vi "ElevatorSim_UpdateX.vi"(8 "dT_Seconds":dbl=1.0, 9 "U":T4, 10 "current_xHat":T4, 11 "ELEVATOR_SIM":T1 {"GearBox"."Kt_NMPerAmp" format="%13.5p"; "GearBox"."Kv_RadPerSecPerVolt" format="%13.5p"; "GearBox"."R_Ohms" format="%13.5p"; "GearBox"."FreeSpeed_RadPerSec" format="%13.5p"; "GearBox"."FreeCurrent_Amps" format="%13.5p"; "GearBox"."StallCurrent_Amps" format="%13.5p"; "GearBox"."StallTorque_NM" format="%13.5p"; "GearBox"."nominalVoltage_Volts" format="%13.5p"}) -> (3 "updated_xHat":T4)   [LabVIEW 2019, in "Trajectory_Library.lvlib"]
doc: "Creates a new LINEAR SYSTEM data cluster with the specified values. \n\n\nInputs: \n - XXX -- XXX.\n\nOutputs:\n - XXX -- XXX."
uses:
  Trajectory_Library.lvlib
  <vilib>/Analysis/Matrix/Datatypes/RealMatrix.ctl
  ELEVATOR_SIM.ctl
  LINEAR_SYSTEM_SIM.ctl
  LINEAR_SYSTEM.ctl
  DCMOTOR.CTL
  MatBuilder_Create.vi
  ElevatorSim_Rkf45_Func.vi
  <vilib>/Analysis/Matrix/NI_Matrix.lvlib
panel:
  # "<States, 1>"
  # "<Outputs, 1>"
  # "<Inputs, 1>"
  # "<Outputs, 1>"
  # "<States,States>"
  # "<States,Inputs>"
  # "<Outputs,States>"
  # "<Outputs,Inputs>"
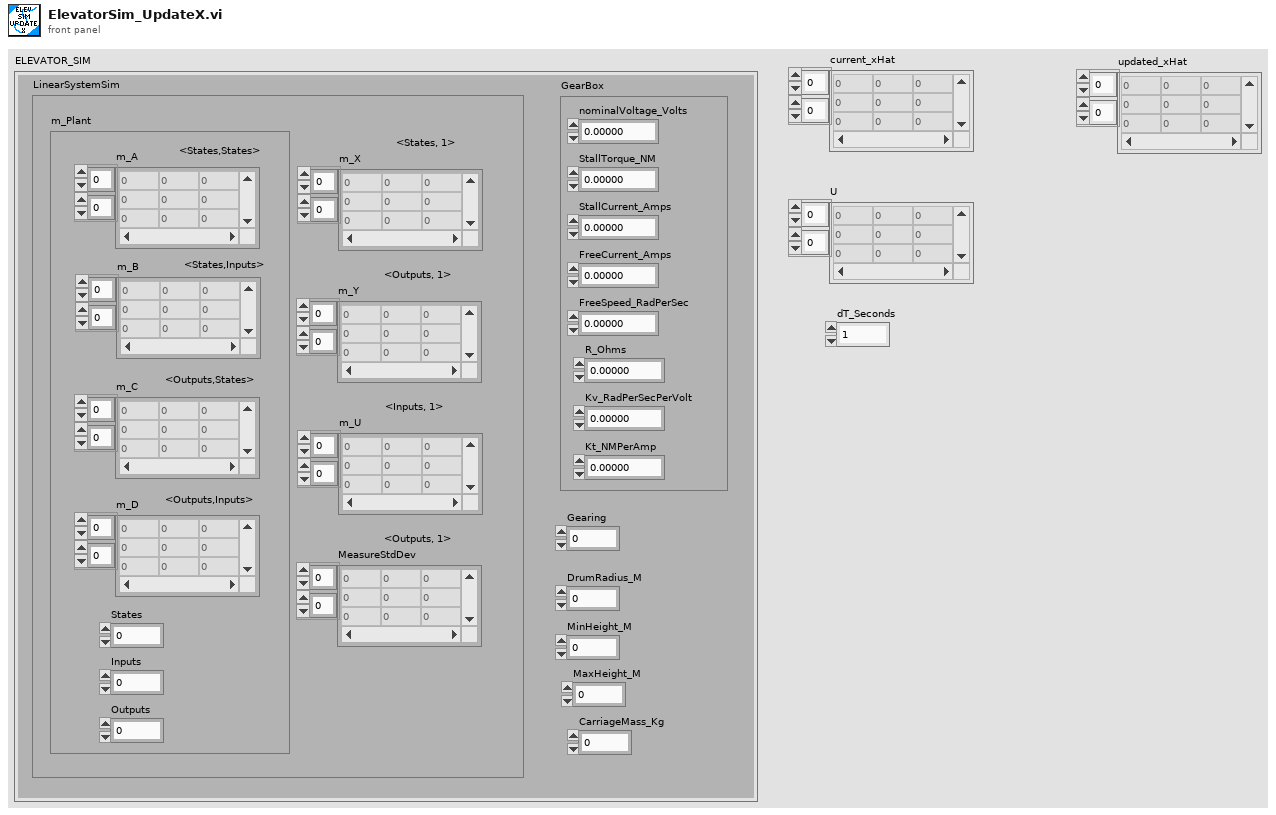
[diagram p1: front panel]
types:
  T1 = typedef "Trajectory_Library.lvlib/ELEVATOR_SIM.ctl" = cluster{"LinearSystemSim":T2, "GearBox":T5, "Gearing":dbl, "DrumRadius_M":dbl, "MinHeight_M":dbl, "MaxHeight_M":dbl, "CarriageMass_Kg":dbl}
  T2 = typedef "Trajectory_Library.lvlib/LINEAR_SYSTEM_SIM.ctl" = cluster{"m_Plant":T3, "m_X":T4, "m_Y":T4, "m_U":T4, "MeasureStdDev":T4}
  T3 = typedef "Trajectory_Library.lvlib/LINEAR_SYSTEM.ctl" = cluster{"m_A":T4, "m_B":T4, "m_C":T4, "m_D":T4, "States":i32, "Inputs":i32, "Outputs":i32}
  T4 = typedef "NI_Matrix.lvlib/RealMatrix.ctl" = dbl[][]
  T5 = typedef "Trajectory_Library.lvlib/DCMOTOR.CTL" = cluster{"nominalVoltage_Volts":dbl, "StallTorque_NM":dbl, "StallCurrent_Amps":dbl, "FreeCurrent_Amps":dbl, "FreeSpeed_RadPerSec":dbl, "R_Ohms":dbl, "Kv_RadPerSecPerVolt":dbl, "Kt_NMPerAmp":dbl}
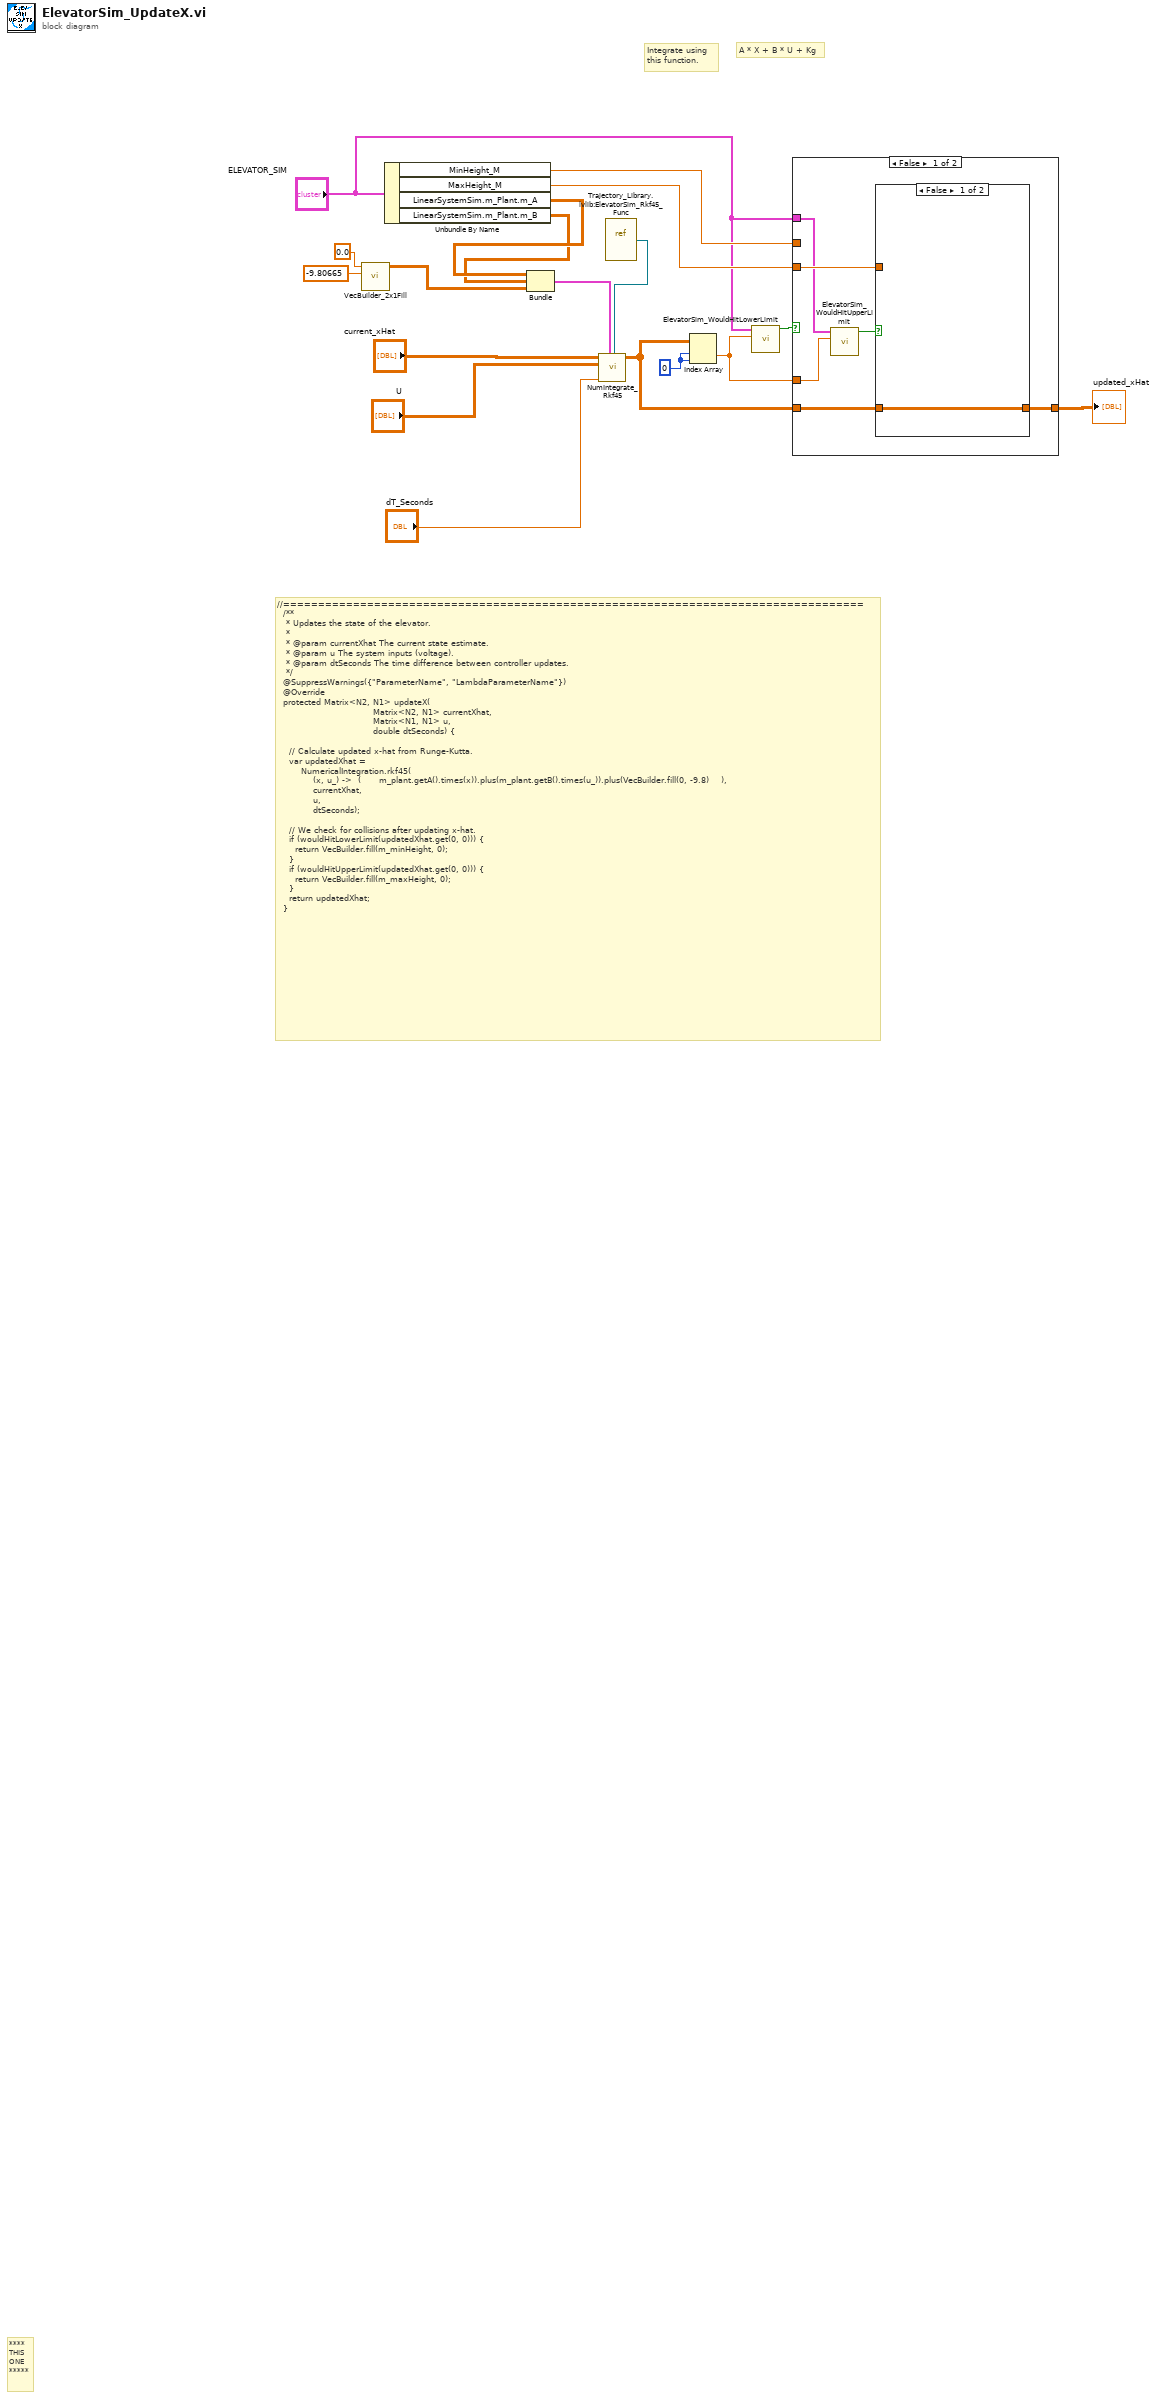
[diagram p0: block diagram]
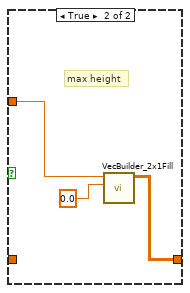
[diagram p2: hidden frame]
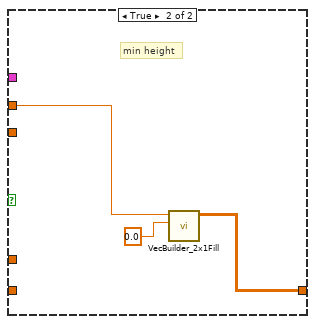
[diagram p3: hidden frame]
diagram:
  w13 = 0 ("index (row)")
  # "Integrate using\nthis function."
  # "A * X + B * U + Kg"
  # "//===================================================================================\n  /**\n   * Updates the state of the elevator.\n   *\n   * @param currentXhat The current state estimate.\n   * @param u The system inputs (voltage).\n   * @param dtSeconds The time difference between controller updates.\n   */\n  @SuppressWarnings({\"ParameterName\", \"LambdaParameterName\"})\n  @Override\n  protected Matrix<N2, N1> updateX(\n                                Matrix<N2, N1> currentXhat, \n                                Matrix<N1, N1> u, \n                                double dtSeconds) {\n\n    // Calculate updated x-hat from Runge-Kutta.\n    var updatedXhat =\n        NumericalIntegration.rkf45(\n            (x, u_) ->  (      m_plant.getA().times(x)).plus(m_plant.getB().times(u_)).plus(VecBuilder.fill(0, -9.8)    ),\n            currentXhat,\n            u,\n            dtSeconds);\n\n    // We check for collisions after updating x-hat.\n    if (wouldHitLowerLimit(updatedXhat.get(0, 0))) {\n      return VecBuilder.fill(m_minHeight, 0);\n    }\n    if (wouldHitUpperLimit(updatedXhat.get(0, 0))) {\n      return VecBuilder.fill(m_maxHeight, 0);\n    }\n    return updatedXhat;\n  }"
  # "****\nTHIS\nONE\n*****"
  n1 = call "VecBuilder_2x1Fill.vi"("R1"=-9.80665, "R0"=0.0) -> ("output matrix"=w3:T4)  [unwired: 9 in]
  n2 = Unbundle By Name("ELEVATOR_SIM") -> ("MinHeight_M"=w7:dbl, "MaxHeight_M"=w12:dbl, "LinearSystemSim.m_Plant.m_A"=w5:T4, "LinearSystemSim.m_Plant.m_B"=w4:T4)
  n3 = Bundle("m_A"=w5, "m_B"=w4, "output matrix"=w3) -> (w2:cluster{"m_A":T4, "m_B":T4, "output matrix":T4})  [unwired: 1 in]
  n4 = vi-ref "Trajectory_Library.lvlib:ElevatorSim_Rkf45_Func.vi"() -> (w1:refnum<vi>)
  n5 = call "NumIntegrate_Rkf45.vi"("NumInt_RKF45_Func_Type"=w1, "PassedData"=w2, "dT_Seconds"="dT_Seconds", "U"="U", "X"="current_xHat") -> ("Return X"=w11:T4)  [unwired: 5 in, 1 out]
  n6 = Index Array(array=w11, index (row)=w13, index (col)=w13) -> (element=w8:dbl)
  n7 = call "ElevatorSim_WouldHitLowerLimit.vi"("ElevHeight_Meters"=w8, "ElevatorSim"="ELEVATOR_SIM") -> ("AtLowLimit"=w9:bool)  [unwired: 9 in]
  n8 = case shown="False" w9 {
    tunnel: w12 -> [w20 _]
    tunnel: w11 -> [w24 _]
    tunnel: [w23 w29] -> w10
    tunnel: w8 -> [w21 _]
    tunnel: w7 -> [_ w30]
    tunnel: "ELEVATOR_SIM" -> [w19 _]
    frame False {
      n9 = call "ElevatorSim_WouldHitUpperLimit.vi"("Height_Meters"=w21, "ElevatorSim"=w19) -> ("At HIgh LImit"=w22:bool)  [unwired: 9 in]
      n10 = case shown="False" w22 {
        tunnel: w24 -> [w25 _]
        tunnel: [w25 w26] -> w23
        tunnel: w20 -> [_ w27]
        frame False {
        }
        frame True {
          # "max height"
          n11 = call "VecBuilder_2x1Fill.vi"("R1"=0.0, "R0"=w27) -> ("output matrix"=w26:T4)  [unwired: 9 in]
        }
      }
    }
    frame True {
      # "min height"
      n12 = call "VecBuilder_2x1Fill.vi"("R1"=0.0, "R0"=w30) -> ("output matrix"=w29:T4)  [unwired: 9 in]
    }
  }
  "updated_xHat" <- w10
